vi "Start Undo.vi"(8 "error in (no error)":errorcluster, 10 "Name":string, 11 "CSM-Helper in":refnum<class "CSM-Helper.lvclass">) -> (0 "error out":errorcluster, 3 "CSM-Helper out":refnum<class "CSM-Helper.lvclass">)   [LabVIEW 2020, in "CSM-Helper.lvclass"]
uses:
  CSM-Helper.lvclass
  CSM-Helper.lvclass/CSM-Helper.ctl
  Properties/Read VI Ref.vi
  <userlib>/_NEVSTOP/Communicable State Machine(CSM)/Communicable State Machine.lvlib
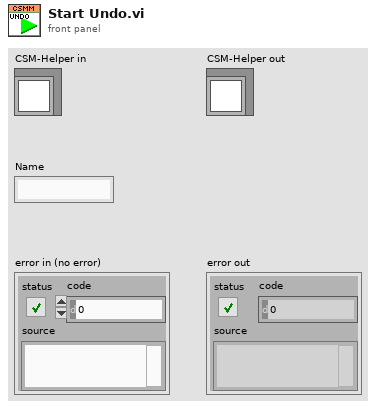
[diagram p1: front panel]
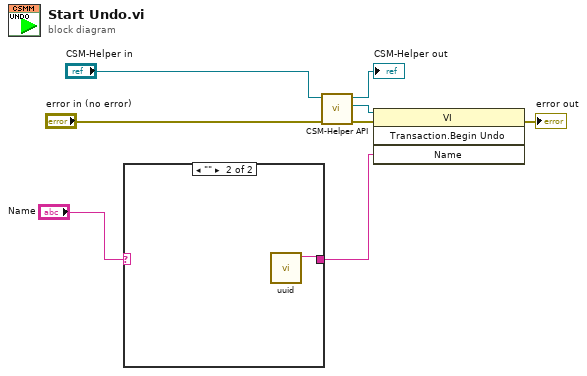
[diagram p0: block diagram]
diagram:
  n1 = case shown="\"\"" "Name" {
    selector: "Name" -> [w9 _]
    tunnel: [w9 w10] -> w1
    frame "False", Default {
    }
    frame "" {
      n2 = call <userlib>:"uuid.vi"() -> ("UUID"=w10:string)  [unwired: 11 in]
    }
  }
  n3 = call-poly "CSM-Helper API.vi"("error in (no error)"="error in (no error)", "CSM-Helper in"="CSM-Helper in") -> ("error out"=w6:errorcluster, "VI"=w8:refnum<vi>, "CSM-Helper out"=→"CSM-Helper out":refnum<class "CSM-Helper.lvclass">)  [unwired: 7 in]
  n4 = invoke class="VI" method="Transaction.Begin Undo"(reference=w8, error in=w6, "Name"=w1) -> (error out=→"error out":errorcluster)  [unwired: 1 in, 3 out]
